vi "Plot Closed.vi"(8 "error in (no error)":errorcluster, 10 "Closed plot":refnum<class "Message Enqueuer.lvclass">, 11 "Application Controller in":refnum<class "Application Controller.lvclass">) -> (0 "error out":errorcluster, 3 "Application Controller out":refnum<class "Application Controller.lvclass">)   [LabVIEW 2016, in "Application Controller.lvclass"]
uses:
  Application Controller.lvclass
  <vilib>/ActorFramework/Message Enqueuer/Message Enqueuer.lvclass
  Application Controller.lvclass/Application Controller.ctl
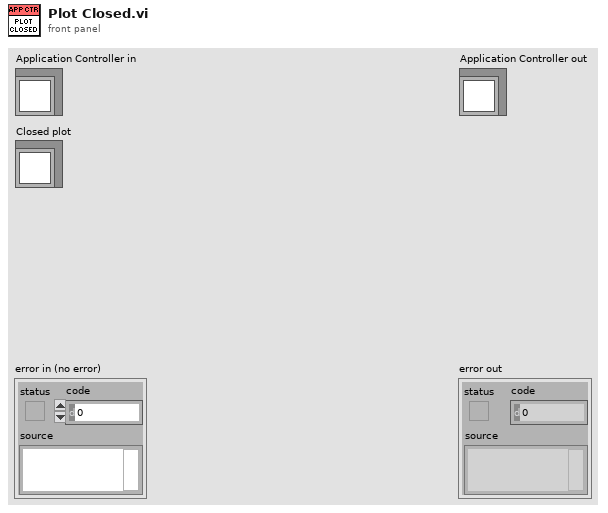
[diagram p1: front panel]
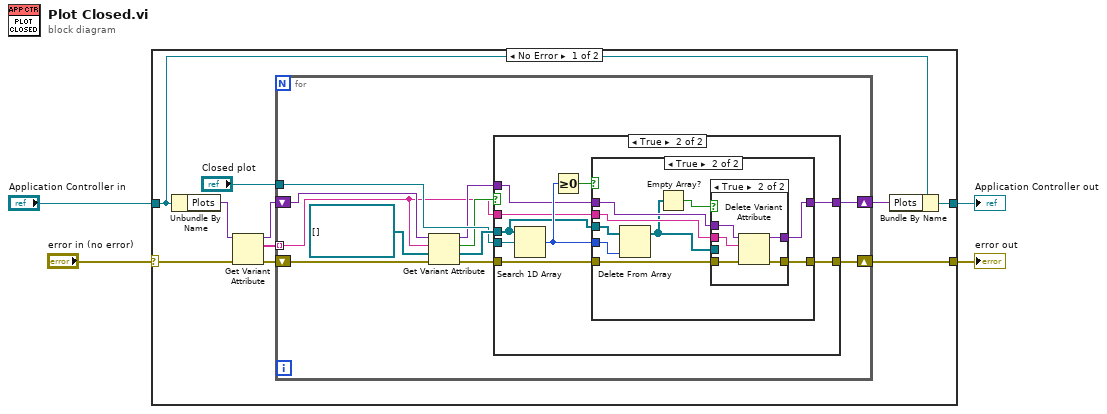
[diagram p0: block diagram]
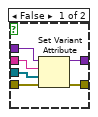
[diagram p4: hidden frame]
diagram:
  n1 = case shown="No Error" "error in (no error)" {
    selector: "error in (no error)" -> [w6 w60]
    tunnel: [w5 w60] -> w3
    tunnel: [w8 w59] -> w1
    tunnel: "Application Controller in" -> [w14 w59]
    frame No Error {
      n2 = Unbundle By Name(w14) -> ("Plots"=w13:variant)
      n3 = Get Variant Attribute(Variant=w13, error in=w6) -> (duplicate Variant=w11:variant, names=w12:string[], error out=w10:errorcluster)  [unwired: 2 in, 1 out]
      n4 = for {
        tunnel: w12 -> [w18] mode=indexing
        shift-right: [w16] -> w5
        shift-left: w10 -> [w24]
        tunnel: "Closed plot" -> [w21]
        shift-right: [w15] -> w7
        shift-left: w11 -> [w25]
        n5 = Get Variant Attribute(Variant=w25, name=w18, default value (empty Variant)=refnum<class "Message Enqueuer.lvclass">[] [] ("Plot enqueuers"), error in=w24) -> (duplicate Variant=w19:variant, found=w20:bool, value=w22:refnum<class "Message Enqueuer.lvclass">[], error out=w17:errorcluster)
        n6 = case shown="True" w20 {
          tunnel: w22 -> [_ w34]
          tunnel: w21 -> [_ w33]
          tunnel: w19 -> [w26 w32]
          tunnel: w18 -> [_ w31]
          tunnel: w17 -> [w27 w30]
          tunnel: [w27 w29] -> w16
          tunnel: [w26 w28] -> w15
          frame False {
          }
          frame True {
            n7 = Search 1D Array(1D array=w34, element=w33) -> (index of element=w35:i32)  [unwired: 1 in]
            n8 = Greater Or Equal To 0?(x=w35) -> (x >= 0?=w36:bool)
            n9 = case shown="True" w36 {
              tunnel: w34 -> [_ w47]
              tunnel: w35 -> [_ w46]
              tunnel: w32 -> [w38 w44]
              tunnel: [w38 w45] -> w28
              tunnel: w31 -> [_ w43]
              tunnel: w30 -> [w37 w42]
              tunnel: [w37 w41] -> w29
              frame False {
              }
              frame True {
                n10 = Delete From Array(array=w47, index=w46) -> (array with subset deleted=w40:refnum<class "Message Enqueuer.lvclass">[])  [unwired: 1 in, 1 out]
                n11 = Empty Array?(array=w40) -> (empty?=w39:bool)
                n12 = case shown="True" w39 {
                  tunnel: [w53 w56] -> w45
                  tunnel: w44 -> [w52 w55]
                  tunnel: w43 -> [w51 w54]
                  tunnel: w42 -> [w50 w58]
                  tunnel: [w49 w57] -> w41
                  tunnel: w40 -> [w48 _]
                  frame False {
                    n13 = Set Variant Attribute(Variant=w52, name=w51, value=w48, error in=w50) -> (Variant out=w53:variant, error out=w49:errorcluster)  [unwired: 1 out]
                  }
                  frame True {
                    n14 = Delete Variant Attribute(4:w58, 6:w54, 7:w55) -> (0:w57:errorcluster, 3:w56:variant)  [unwired: 1 out]
                  }
                }
              }
            }
          }
        }
      }
      n15 = Bundle By Name(cluster=w14, "Plots"=w7) -> (w8:refnum<class "Application Controller.lvclass">)
    }
    frame Error {
    }
  }
  "error out" <- w3
  "Application Controller out" <- w1
